vi "LoggingTesting.vi"() -> ()   [LabVIEW 2018]
doc: "A simple VI to test logging. Logs to TestLog.csv in the Robot-Project/Logging/ folder."
uses:
  LogOperation.ctl
  DataNames.ctl
panel:
  in  "Boolean":bool=TRUE
  in  "Numeric":dbl=1.0 format="%#_13g"
  in  "Hello":string="Apple"
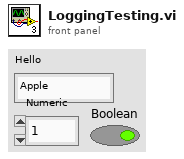
[diagram p1: front panel]
types:
  T1 = typedef "LogOperation.ctl" = enum16{"Set", "Get All", "Get Headers"}
  T2 = enum16{"open", "replace", "create", "open or create", "replace or create", "replace or create with confirmation"}
  T3 = typedef "DataNames.ctl" = enum16{"RobotMode", "FMSConnected", "DriveLeft", "DriveRight", "EncoderLeft", "EncoderRight", "Angle", "LocationX", "LocationY", "CPU", "DriveOperation", "Battery"}
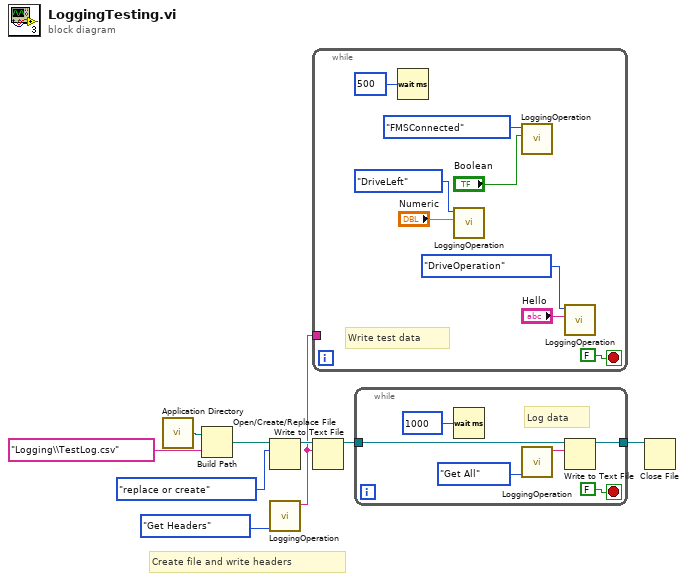
[diagram p0: block diagram]
diagram:
  # "Create file and write headers"
  n1 = call <vilib>:"Application Directory.vi"() -> ("Application Directory"=w5:path)
  n2 = Build Path(base path=w5, name or relative path="Logging\\TestLog.csv") -> (appended path=w4:path)
  n3 = Open/Create/Replace File(file path (use dialog)=w4, operation (0:open)=T2."replace or create") -> (refnum out=w9:refnum<file>)  [unwired: 4 in, 2 out]
  n4 = call "LoggingOperation.vi"("Operation"=LogOperation."Get Headers") -> ("Log String"=w1:string)  [unwired: 10 in]
  n5 = while {
    tunnel: w1 -> [_]
    stop <- FALSE stop-if-true
    # "Write test data"
    n6 = Wait (ms)(milliseconds to wait=u32 500) -> ()  [unwired: 1 out]
    n7 = call "LoggingOperation.vi"("Data"="Numeric", "Name"=DataNames."DriveLeft") -> ()  [unwired: 9 in, 1 out]
    n8 = call "LoggingOperation.vi"("Data"="Boolean", "Name"=DataNames."FMSConnected") -> ()  [unwired: 9 in, 1 out]
    n9 = call "LoggingOperation.vi"("Data"="Hello", "Name"=DataNames."DriveOperation") -> ()  [unwired: 9 in, 1 out]
  }
  n10 = Write to Text File(file (use dialog)=w9, text=w1) -> (refnum out=w7:refnum<file>)  [unwired: 2 in, 2 out]
  n11 = while {
    tunnel: w7 -> [w20]
    tunnel: [w19] -> w6
    stop <- FALSE stop-if-true
    # "Log data"
    n12 = Wait (ms)(milliseconds to wait=u32 1000) -> ()  [unwired: 1 out]
    n13 = call "LoggingOperation.vi"("Operation"=LogOperation."Get All") -> ("Log String"=w18:string)  [unwired: 10 in]
    n14 = Write to Text File(file (use dialog)=w20, text=w18) -> (refnum out=w19:refnum<file>)  [unwired: 2 in, 2 out]
  }
  n15 = Close File(refnum=w6) -> ()  [unwired: 1 in, 2 out]
